vi "DQMH Configure (Cloneable).vi"(7 "Module Disk Path":path, 8 "error in (no error)":errorcluster, 11 "Application reference":refnum<vi>) -> (0 "error out":errorcluster)   [LabVIEW 2022 SP3, in "hse-dqmh-dynamicrequesters.lvlib"]
doc: "Calls the \"Configure\" request VI of the module in <b>path</b>\n\n____\nHAMPEL SOFTWARE ENGINEERING v3.8.0 (2023-12-18 14:41)"
uses:
  hse-dqmh-dynamicrequesters.lvlib
panel:
  in  "Module ID":i32
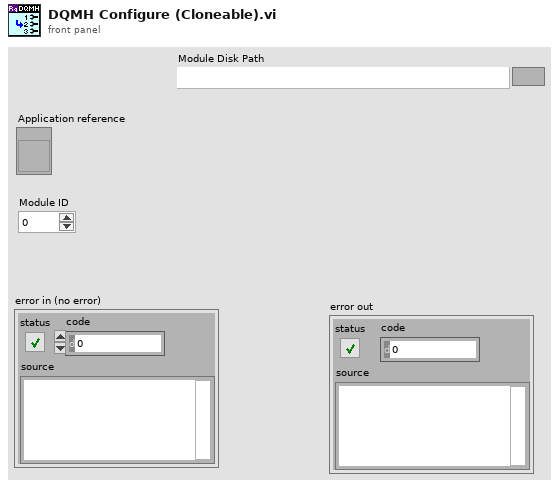
[diagram p1: front panel]
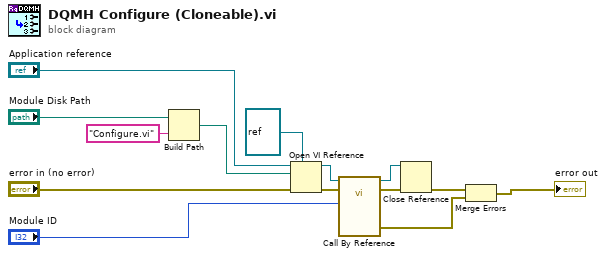
[diagram p0: block diagram]
diagram:
  n1 = Build Path(base path="Module Disk Path", name or relative path="Configure.vi") -> (appended path=w3:path)
  n2 = Open VI Reference(type specifier VI Refnum (for type only)=refnum<vi> refnum, application reference (local)="Application reference", vi path=w3, error in (no error)="error in (no error)") -> (vi reference=w4:refnum<vi>, error out=w5:errorcluster)  [unwired: 2 in]
  n3 = call-by-ref "?"(reference=w4, error in=w5, "Module ID"="Module ID") -> (reference out=w10:refnum<vi>, error out=w9:errorcluster, 0:"error out"=w12:errorcluster)  [unwired: 10 in]
  n4 = Close Reference(reference=w10, error in (no error)=w9) -> (error out=w8:errorcluster)
  n5 = Merge Errors(w8, w12) -> (→"error out":errorcluster)
